vi "Load Config INI from Filename.vi"(6 "File Name":string, 7 "File Type":string(combo)=".gif", 8 "Error In":errorcluster, 10 "reference":refnum<vi>, 11 "Path In":path) -> (0 "Error Out":errorcluster, 3 "Path Out":path)   [LabVIEW 2015]
uses:
  <vilib>/Utility/config.llb/Read Key (String).vi
  <vilib>/Utility/config.llb/NI_LVConfig.lvlib
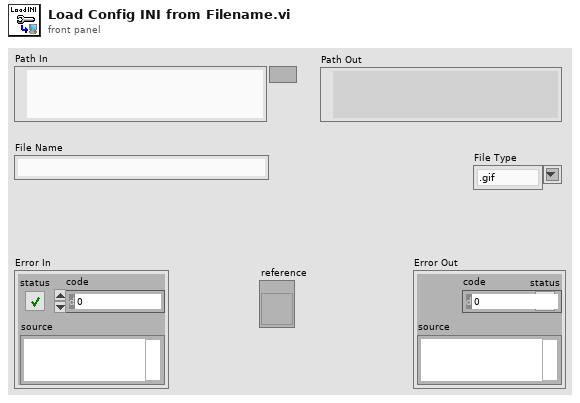
[diagram p1: front panel]
types:
  T1 = typedef "NI_LVConfig.lvlib/Config Data RefNum.ctl" = refnum<k1>
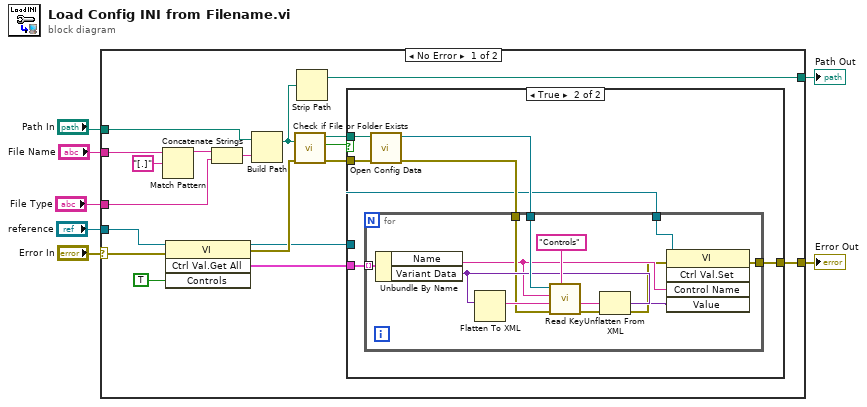
[diagram p0: block diagram]
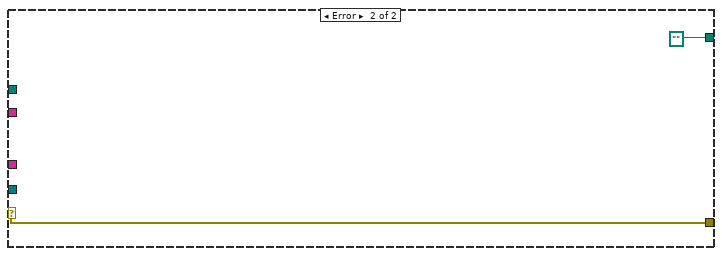
[diagram p3: hidden frame]
diagram:
  n1 = case shown="No Error" "Error In" {
    selector: "Error In" -> [w19 w48]
    tunnel: [w15 w48] -> w5
    tunnel: [w8 path ""] -> w4
    tunnel: "Path In" -> [w11 _]
    tunnel: "reference" -> [w13 _]
    tunnel: "File Type" -> [w12 _]
    tunnel: "File Name" -> [w10 _]
    frame No Error {
      n2 = Match Pattern(string=w10, regular expression="[.]" ("search string")) -> (before substring=w24:string)  [unwired: 1 in, 3 out]
      n3 = invoke class="VI" method="Ctrl Val.Get All"(reference=w13, error in=w19, "Controls"=TRUE) -> (reference out=w16:refnum<vi>, error out=w18:errorcluster, "Get All Control Values Variant"=w17:cluster{"Name":string, "Variant Data":variant}[])  [unwired: 1 in, 1 out]
      n4 = Concatenate Strings(w24, w12) -> (w23:string)
      n5 = Build Path(base path=w11, name or relative path=w23) -> (appended path=w9:path)
      n6 = call <vilib>:"Check if File or Folder Exists.vi"("error in (no error)"=w18, "path"=w9) -> ("error out"=w21:errorcluster, "file or folder exists?"=w22:bool, "dup path"=w14:path)  [unwired: 7 in]
      n7 = Strip Path(path=w9) -> (stripped path=w8:path)  [unwired: 1 out]
      n8 = case shown="True" w22 {
        tunnel: w14 -> [_ w33]
        tunnel: w21 -> [w26 w32]
        tunnel: w17 -> [_ w31]
        tunnel: w16 -> [_ w28]
        tunnel: [w26 w27] -> w15
        frame False {
        }
        frame True {
          n9 = call <vilib>:"Open Config Data.vi"("error in (no error)"=w32, "configuration file path"=w33) -> ("error out"=w29:errorcluster, "refnum"=w30:T1)  [unwired: 1 in, 7 out]
          n10 = for {
            tunnel: w31 -> [w45] mode=indexing
            tunnel: w30 -> [w44]
            tunnel: w29 -> [w40]
            tunnel: w28 -> [w38]
            tunnel: [w34] -> w27
            n11 = Unbundle By Name(w45) -> ("Name"=w37:string, "Variant Data"=w42:variant)
            n12 = Flatten To XML(anything=w42) -> (xml string=w43:string)
            n13 = call-poly <vilib>:"Read Key.vi"("section"="Controls", "error in (no error)"=w40, "default value"=w43, "key"=w37, "refnum"=w44) -> ("error out"=w39:errorcluster, "value"=w41:string)  [unwired: 3 in, 2 out]
            n14 = Unflatten From XML(xml string=w41, type=w42, error in (no error)=w39) -> (value=w36:variant, error out=w35:errorcluster)
            n15 = invoke class="VI" method="Ctrl Val.Set"(reference=w38, error in=w35, "Control Name"=w37, "Value"=w36) -> (error out=w34:errorcluster)  [unwired: 1 in, 4 out]
          }
        }
      }
    }
    frame Error {
      (unwired) ""
    }
  }
  "Error Out" <- w5
  "Path Out" <- w4
